vi "低层函数-Ring.vi"() -> ()   [LabVIEW 2018]
uses:
  <vilib>/userdefined/High Color/IMAQdx.ctl
  <vilib>/vision/Image Controls.llb/IMAQ Image.ctl
  <vilib>/vision/driver/IMAQdx.llb/IMAQdx Acquisition Mode.ctl
  <vilib>/vision/driver/IMAQdx.llb/IMAQdx Buffer Number Mode.ctl
  <vilib>/vision/driver/NI_Vision_Acquisition_Software.lvlib
panel:
  out "数组":T1[](array[typedef])
  in  "Number of Buffers":u32=1
  in  "布尔":bool
  out "error out":errorcluster
  out "Image":T1(plugin-control)
  in  "error in":errorcluster
  in  "Session In":T2
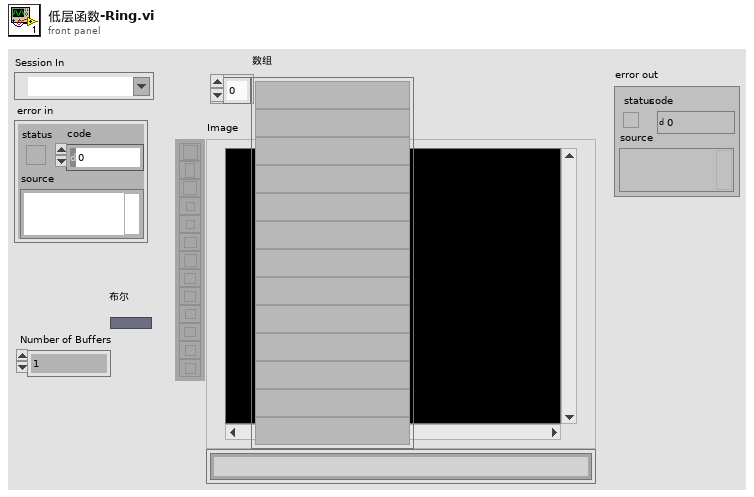
[diagram p1: front panel]
types:
  T1 = typedef "IMAQ Image.ctl" = refnum<image>
  T2 = typedef "IMAQdx.ctl" = refnum<k21>
  T3 = typedef "NI_Vision_Acquisition_Software.lvlib/IMAQdx Acquisition Mode.ctl" = enum32{"One Shot", "Continuous"}
  T4 = typedef "NI_Vision_Acquisition_Software.lvlib/IMAQdx Buffer Number Mode.ctl" = enum32{"Next", "Last", "Buffer Number", "Every", "Last New"}
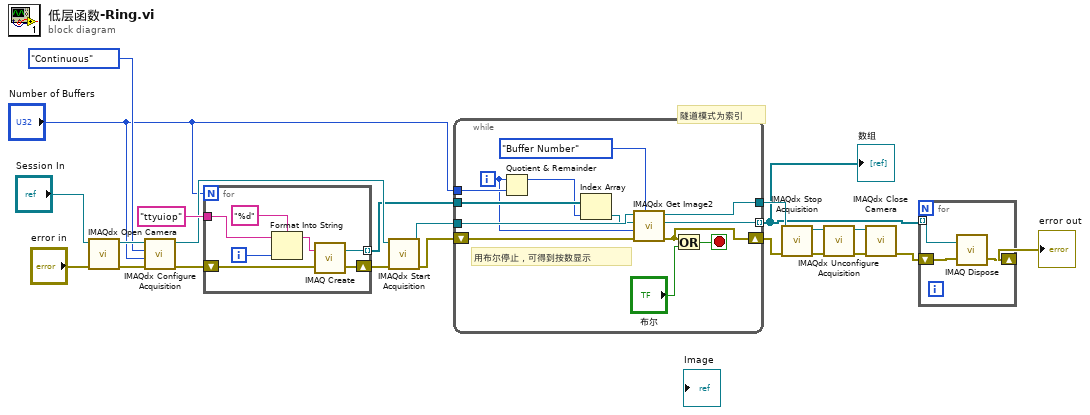
[diagram p0: block diagram]
diagram:
  # "隧道模式为索引"
  n1 = call <vilib>:"IMAQdx Open Camera.vi"("error in"="error in", "Session In"="Session In") -> ("error out"=w18:errorcluster, "Session Out"=w21:T2)  [unwired: 8 in]
  n2 = call <vilib>:"IMAQdx Configure Acquisition.vi"("error in"=w18, "Number of Buffers"="Number of Buffers", "Continuous?"=IMAQdx_Acquisition_Mode."Continuous", "Session In"=w21) -> ("error out"=w22:errorcluster, "Session Out"=w4:T2)  [unwired: 6 in]
  n3 = for {
    N: "Number of Buffers" -> [_]
    shift-right: [w28] -> w17
    shift-left: w22 -> [w29]
    tunnel: "ttyuiop" ("初始字符串") -> [w25]
    tunnel: [w23] -> w2 mode=indexing
    i -> [w27]
    n4 = Format Into String(format string="%d" ("格式字符串"), initial string=w25, w27) -> (resulting string=w24:string)  [unwired: 1 in, 1 out]
    n5 = call "IMAQ Create"("Image Name"=w24, "error in (no error)"=w29) -> ("New Image"=w23:T1, "error out"=w28:errorcluster)  [unwired: 3 in]
  }
  n6 = call <vilib>:"IMAQdx Start Acquisition.vi"("error in"=w17, "Session In"=w4) -> ("error out"=w12:errorcluster, "Session Out"=w13:T2)  [unwired: 8 in]
  n7 = while {
    tunnel: w13 -> [w36]
    tunnel: [w40] -> w10
    shift-right: [w38] -> w11
    shift-left: w12 -> [w42]
    tunnel: "Number of Buffers" -> [w31]
    tunnel: w2 -> [w35]
    tunnel: [w32] -> w1 mode=indexing
    i -> [w30]
    stop <- w37 stop-if-true
    # "用布尔停止，可得到按数显示"
    n8 = Quotient & Remainder(x=w30, y=w31) -> (x-y*floor(x/y)=w34:u32)  [unwired: 1 out]
    n9 = Index Array(array=w35, index=w34) -> (element=w33:T1)
    n10 = call <vilib>:"IMAQdx Get Image2.vi"("Buffer Number Mode (Next)"=IMAQdx_Buffer_Number_Mode."Buffer Number", "error in"=w42, "Buffer Number In"=w30, "Image In"=w33, "Session In"=w36) -> ("error out"=w38:errorcluster, "Image Out"=w32:T1, "Session Out"=w40:T2)  [unwired: 3 in, 1 out]
    n11 = Or(x=w38, y="布尔") -> (x .or. y?=w37:bool)
  }
  "数组" <- w1
  n12 = call <vilib>:"IMAQdx Stop Acquisition.vi"("error in"=w11, "Session In"=w10) -> ("error out"=w8:errorcluster, "Session Out"=w9:T2)  [unwired: 8 in]
  n13 = call <vilib>:"IMAQdx Unconfigure Acquisition.vi"("error in"=w8, "Session In"=w9) -> ("error out"=w6:errorcluster, "Session Out"=w7:T2)  [unwired: 8 in]
  n14 = call <vilib>:"IMAQdx Close Camera.vi"("error in"=w6, "Session In"=w7) -> ("error out"=w15:errorcluster)  [unwired: 9 in]
  n15 = for {
    shift-right: [w44] -> w14
    shift-left: w15 -> [w45]
    tunnel: w1 -> [w43] mode=indexing
    n16 = call "IMAQ Dispose"("Image"=w43, "error in (no error)"=w45) -> ("error out"=w44:errorcluster)  [unwired: 4 in]
  }
  "error out" <- w14
